vi "SYST_COMM_GPIB_RDEV_RES.vi"(0 "VISA IN":refnum<visa-resource-name>, 5 "error in":errorcluster) -> (14 "VISA Out":refnum<visa-resource-name>, 19 "error out":errorcluster)   [LabVIEW 2018, in "PNA-X.lvlib"]
doc: "SYSTem:COMMunicate:GPIB:RDEVice:RESet \n(Write-only) Performs the same function as SYST:COMM:GPIB:RDEV:CLOS except that ALL \npass-through sessions are closed. \nExamples SYST:COMM:GPIB:RDEV:RES \nQuery Syntax Not Applicable \nDefault Not Applicable"
uses:
  PNA-X.lvlib
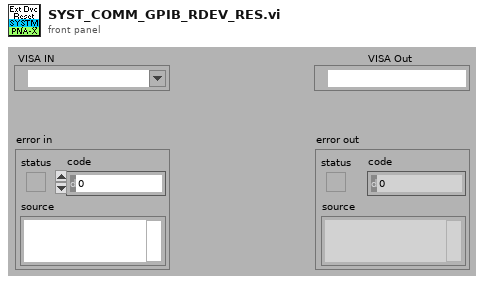
[diagram p1: front panel]
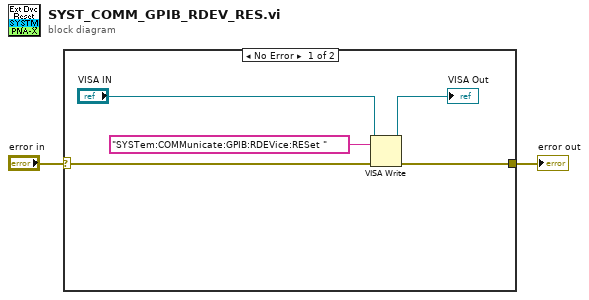
[diagram p0: block diagram]
diagram:
  n1 = case shown="No Error" "error in" {
    selector: "error in" -> [w3 w8]
    tunnel: [w6 w8] -> w1
    frame No Error {
      n2 = VISA Write(VISA resource name="VISA IN", write buffer="SYSTem:COMMunicate:GPIB:RDEVice:RESet " ("Cmdline"), error in (no error)=w3) -> (VISA resource name out=→"VISA Out":refnum<visa-resource-name>, error out=w6:errorcluster)  [unwired: 1 out]
    }
    frame Error {
    }
  }
  "error out" <- w1
